vi "De-spiked_Stats.vi"(0 "Raw Signal":dbl[](array[numeric]), 1 "No of st dev to chop at":dbl=6.0) -> (2 "mean":dbl format="%0.2f", 3 "standard deviation":dbl format="%0.2f", 4 "variance":dbl format="%0.2f")   [LabVIEW 2010]
uses:
  <vilib>/Analysis/NI_AALBase.lvlib
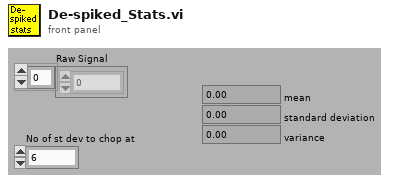
[diagram p1: front panel]
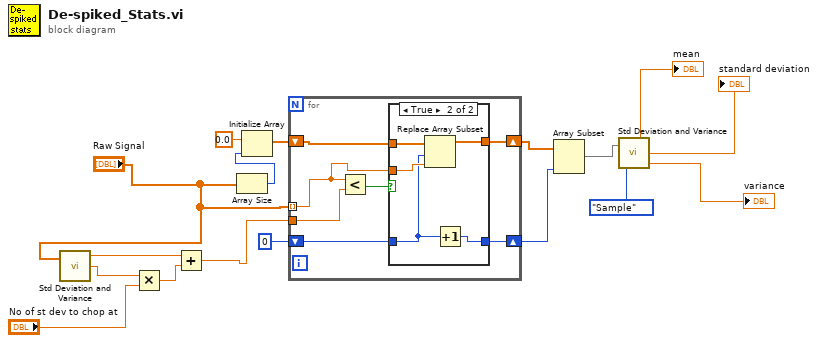
[diagram p0: block diagram]
diagram:
  n1 = call <vilib>:"Std Deviation and Variance.vi"("X"="Raw Signal") -> ("mean"=w13:dbl, "standard deviation"=w12:dbl)  [unwired: 1 in, 1 out]
  n2 = Multiply(x=w12, y="No of st dev to chop at") -> (x*y=w11:dbl)
  n3 = Add(x=w13, y=w11) -> (x+y=w10:dbl)
  n4 = Array Size(array="Raw Signal") -> (size(s)=w17:i32)
  n5 = Initialize Array(0.0 ("element"), w17) -> (w15:dbl[])
  n6 = for {
    shift-right: [w23] -> w9
    shift-left: w15 -> [w24]
    shift-right: [w18] -> w8
    shift-left: 0 -> [w19]
    tunnel: w10 -> [w22]
    tunnel: "Raw Signal" -> [w20] mode=indexing
    n7 = Less?(x=w20, y=w22) -> (x < y?=w21:bool)
    n8 = case shown="True" w21 {
      tunnel: w24 -> [w25 w31]
      tunnel: [w25 w30] -> w23
      tunnel: w20 -> [_ w29]
      tunnel: w19 -> [w26 w28]
      tunnel: [w26 w27] -> w18
      frame False {
      }
      frame True {
        n9 = Replace Array Subset(array=w31, new element=w29, index=w28) -> (w30:dbl[])
        n10 = Increment(x=w28) -> (x+1=w27:i32)
      }
    }
  }
  n11 = Array Subset(array=w9, length=w8) -> (w6:dbl[])  [unwired: 1 in]
  n12 = call <vilib>:"Std Deviation and Variance.vi"("X"=w6, "Weighting (Sample)"=enum16{"Sample", "Population"}."Sample") -> ("mean"=→"mean":dbl, "standard deviation"=→"standard deviation":dbl, "variance"=→"variance":dbl)
